vi "NOR-and-NAND-gates.vi"() -> ()   [LabVIEW 2025]
panel:
  out "Boolean 6":bool
  out "Boolean 5":bool
  in  "Boolean 4":bool
  in  "Boolean 3":bool
  in  "Boolean 2":bool
  in  "Boolean":bool
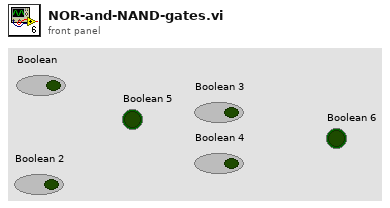
[diagram p1: front panel]
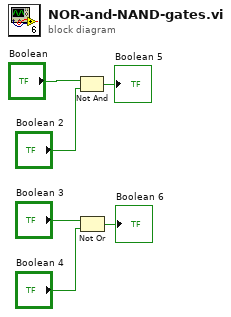
[diagram p0: block diagram]
diagram:
  n1 = Not And(1:"Boolean 2", 2:"Boolean") -> (0:→"Boolean 5":bool)
  n2 = Not Or(1:"Boolean 4", 2:"Boolean 3") -> (0:→"Boolean 6":bool)
